vi "sensores.vi"() -> ()   [LabVIEW 2020]
panel:
  out "Sensores":T1
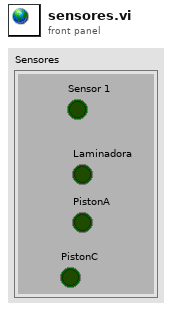
[diagram p1: front panel]
types:
  T1 = cluster{"Sensor 1":bool, "Laminadora":bool, "PistonA":bool, "PistonC":bool}
diagram:
